vi "Write Error.vi"(10 "Error":errorcluster, 11 "Error in":refnum<class "Error.lvclass">) -> (3 "Error out":refnum<class "Error.lvclass">)   [LabVIEW 2021, in "jettl.lvlib" / "Error.lvclass"]
uses:
  Error.lvclass
  Error.lvclass/Error.ctl
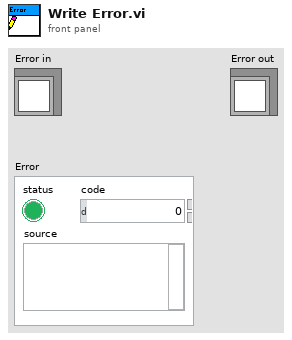
[diagram p1: front panel]
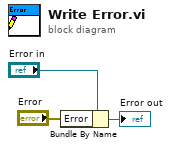
[diagram p0: block diagram]
diagram:
  n1 = Bundle By Name(cluster="Error in", "Error"="Error") -> (→"Error out":refnum<class "Error.lvclass">)
